vi "Check for Flow Cali.vi"(8 "error in (no error)":errorcluster, 10 "Flow array available?":bool, 11 "Flow Array in":dbl[](array[numeric])) -> (0 "error out":errorcluster, 3 "Flow Array out":dbl[](array[numeric]))   [LabVIEW 2020, in "CollectionSupport.lvlib"]
uses:
  CollectionSupport.lvlib
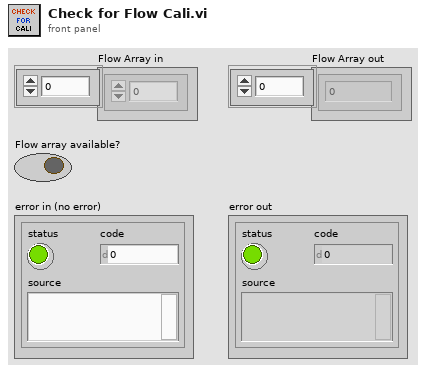
[diagram p1: front panel]
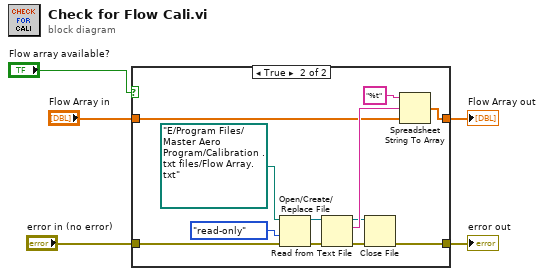
[diagram p0: block diagram]
diagram:
  n1 = case shown="True" "Flow array available?" {
    tunnel: "Flow Array in" -> [w7 w14]
    tunnel: [w7 w17] -> w3
    tunnel: [w6 w13] -> w4
    tunnel: "error in (no error)" -> [w6 w12]
    frame False {
    }
    frame True {
      n2 = Open/Create/Replace File(file path (use dialog)=path "E:/Program Files/Master Aero Program/Calibration .txt files/Flow Array.txt", error in=w12, access (0:read/write)=enum16{"read/write", "read-only", "write-only"}."read-only") -> (refnum out=w10:refnum<file>, error out=w18:errorcluster)  [unwired: 3 in, 1 out]
      n3 = Read from Text File(file (use dialog)=w10, error in=w18) -> (refnum out=w11:refnum<file>, text=w16:string, error out=w19:errorcluster)  [unwired: 2 in, 1 out]
      n4 = Close File(refnum=w11, error in=w19) -> (error out=w13:errorcluster)  [unwired: 1 out]
      n5 = Spreadsheet String To Array(format string="%t", spreadsheet string=w16, array type (2D Dbl)=w14) -> (array=w17:dbl[])  [unwired: 1 in]
    }
  }
  "error out" <- w4
  "Flow Array out" <- w3
